vi "Limit Duty Cycle Range.vi"(0 "duty cycle (scaled) in":u32, 7 "frequency (scaled)":u32, 11 "error in (no error)":errorcluster) -> (4 "duty cycle (scaled) out":u32, 15 "error out":errorcluster)   [LabVIEW 2017, in "NI_FpgaMspHost.lvlib"]
doc: "Limits range of non-zero duty cycles requestable for a given frequency by taking into account the sample period implied by <B>frequency (scaled)</B>."
uses:
  <vilib>/rvi/Analysis/host/Public/NI_FpgaMspHost.lvlib
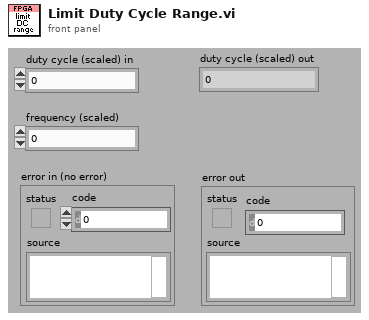
[diagram p1: front panel]
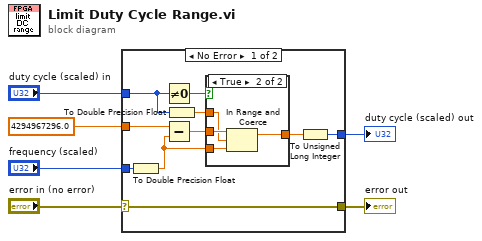
[diagram p0: block diagram]
diagram:
  n1 = case shown="No Error" "error in (no error)" {
    selector: "error in (no error)" -> [w7 w23]
    tunnel: "frequency (scaled)" -> [w15 _]
    tunnel: "duty cycle (scaled) in" -> [w14 w22]
    tunnel: 4294967296.0 ("x") -> [w12 _]
    tunnel: [w10 w22] -> w3
    tunnel: [w7 w23] -> w1
    frame No Error {
      n2 = To Double Precision Float(number=w15) -> (double precision float=w16:dbl)
      n3 = Not Equal To 0?(x=w14) -> (x != 0?=w13:bool)
      n4 = Subtract(x=w12, y=w16) -> (x-y=w11:dbl)
      n5 = To Double Precision Float(number=w14) -> (double precision float=w8:dbl)
      n6 = case shown="True" w13 {
        tunnel: w11 -> [_ w21]
        tunnel: w16 -> [_ w20]
        tunnel: w8 -> [w17 w19]
        tunnel: [w17 w18] -> w9
        frame False {
        }
        frame True {
          n7 = In Range and Coerce(upper limit=w21, x=w19, lower limit=w20) -> (coerced(x)=w18:dbl)  [unwired: 1 out]
        }
      }
      n8 = To Unsigned Long Integer(number=w9) -> (unsigned 32bit integer=w10:u32)
    }
    frame Error {
    }
  }
  "duty cycle (scaled) out" <- w3
  "error out" <- w1
